vi "Calculo_AH.vi"(3 "AH_Telescopio":dbl format="%#.12g", 4 "RA_Destino":dbl format="%#.12g", 5 "Hora Sideral":dbl format="%#.12g") -> (0 "Dif_AH":dbl format="%.9g", 1 "Dif_Abs_AH":dbl format="%.9g", 2 "AH_Destino":dbl format="%.9g")   [LabVIEW 2012]
panel:
  # "-"
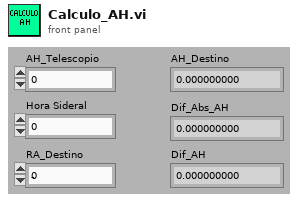
[diagram p1: front panel]
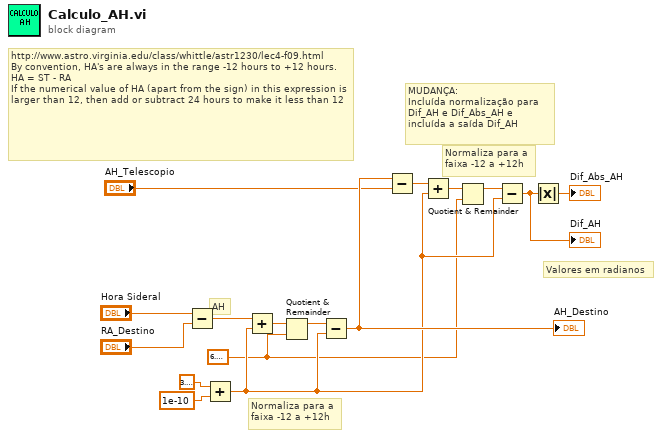
[diagram p0: block diagram]
diagram:
  w2 = 6.283185307179586
  # "MUDANÇA:\nIncluída normalização para \nDif_AH e Dif_Abs_AH e \nincluída a saída Dif_AH"
  # "Normaliza para a\nfaixa -12 a +12h"
  # "AH"
  # "Valores em radianos"
  # "Normaliza para a\nfaixa -12 a +12h"
  # "http://www.astro.virginia.edu/class/whittle/astr1230/lec4-f09.html\nBy convention, HA's are always in the range -12 hours to +12 hours.\nHA = ST - RA\nIf the numerical value of HA (apart from the sign) in this expression is larger than 12, then add or subtract 24 hours to make it less than 12"
  n1 = Subtract(x="Hora Sideral", y="RA_Destino") -> (x-y=w9:dbl)
  n2 = Add(x=3.141592653589793, y=1e-10) -> (x+y=w3:dbl)
  n3 = Add(x=w9, y=w3) -> (x+y=w14:dbl)
  n4 = Quotient & Remainder(x=w14, y=w2) -> (x-y*floor(x/y)=w13:dbl)  [unwired: 1 out]
  n5 = Subtract(x=w13, y=w3) -> (x-y=w5:dbl)
  "AH_Destino" <- w5
  n6 = Subtract(x=w5, y="AH_Telescopio") -> (x-y=w8:dbl)
  n7 = Add(x=w8, y=w3) -> (x+y=w6:dbl)
  n8 = Quotient & Remainder(x=w6, y=w2) -> (x-y*floor(x/y)=w7:dbl)  [unwired: 1 out]
  n9 = Subtract(x=w7, y=w3) -> (x-y=w1:dbl)
  "Dif_AH" <- w1
  n10 = Absolute Value(x=w1) -> (abs(x)=→"Dif_Abs_AH":dbl)
